vi "Create DVR.vi"(8 "Error In":errorcluster, 11 "Arithmetic Class":refnum<class "Arithemetic Operation.lvclass">) -> (0 "Error Out":errorcluster, 3 "DVR":refnum<data-value>)   [LabVIEW 2023, in "Arithemetic Operation.lvclass"]
doc: "The method creates a DVR for the given class data."
uses:
  Arithemetic Operation.lvclass
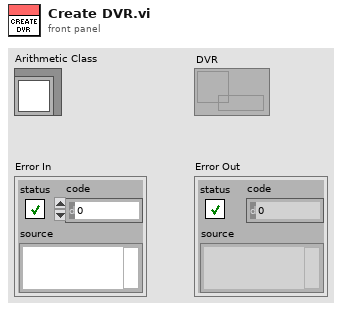
[diagram p1: front panel]
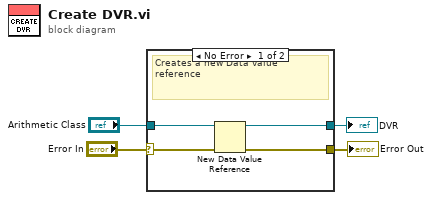
[diagram p0: block diagram]
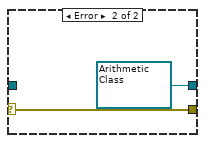
[diagram p2: hidden frame]
diagram:
  n1 = case shown="No Error" "Error In" {
    selector: "Error In" -> [w6 w10]
    tunnel: [w5 w10] -> w3
    tunnel: "Arithmetic Class" -> [w8 _]
    tunnel: [w7 refnum<data-value> refnum ("data value reference")] -> w1
    frame No Error {
      # "Creates a new Data value reference"
      n2 = New Data Value Reference(data value=w8, error in=w6) -> (data value reference=w7:refnum<data-value>, error out=w5:errorcluster)
    }
    frame Error {
    }
  }
  "Error Out" <- w3
  "DVR" <- w1
